vi "Set Up Dialog - Pulse.vi"() -> ()   [LabVIEW 2012]
panel:
  out "Calibration Instructions":string="1. Connect the sensor to your myDAQ as shown in the diagram above.\n\n2. Wrap the pulse sensor very snuggly around your finger with the white pad on the pad of your finger tip. You can try different fingers if the signal is not clear.\n\n3. Wait until the signal has settled then clear the chart and press \"RescaleY\" to scale the data on the chart. You should see distinct spikes with each heartbeat as pictured in Fig 1. Be patient and try to move your hand as little as possible to get a clear signal.\n\n4. Press the Calibrate button to automatically set the threshold limit to 60% of the range of the signal. You can type in your own value for the threshold if needed so that the pulse signal crosses the threshold only once per beat.\n"
  # "iWorx - Pulse - Set Up"
  # "Fig 1. Example Waveform Chart form the Pulse Data Logger VI"
  # "Pulse Sensor (PTN - 104)"
  # "iWorx"
  # "Sensor"
  # "PTN - 104"
  # "myDAQ"
  # "Computer"
  # "Adaptor"
  # "Connection Diagram"
  # "For this chart the threshold is set to 64uV, so the signal crosses the threashold once ber heartbeat."
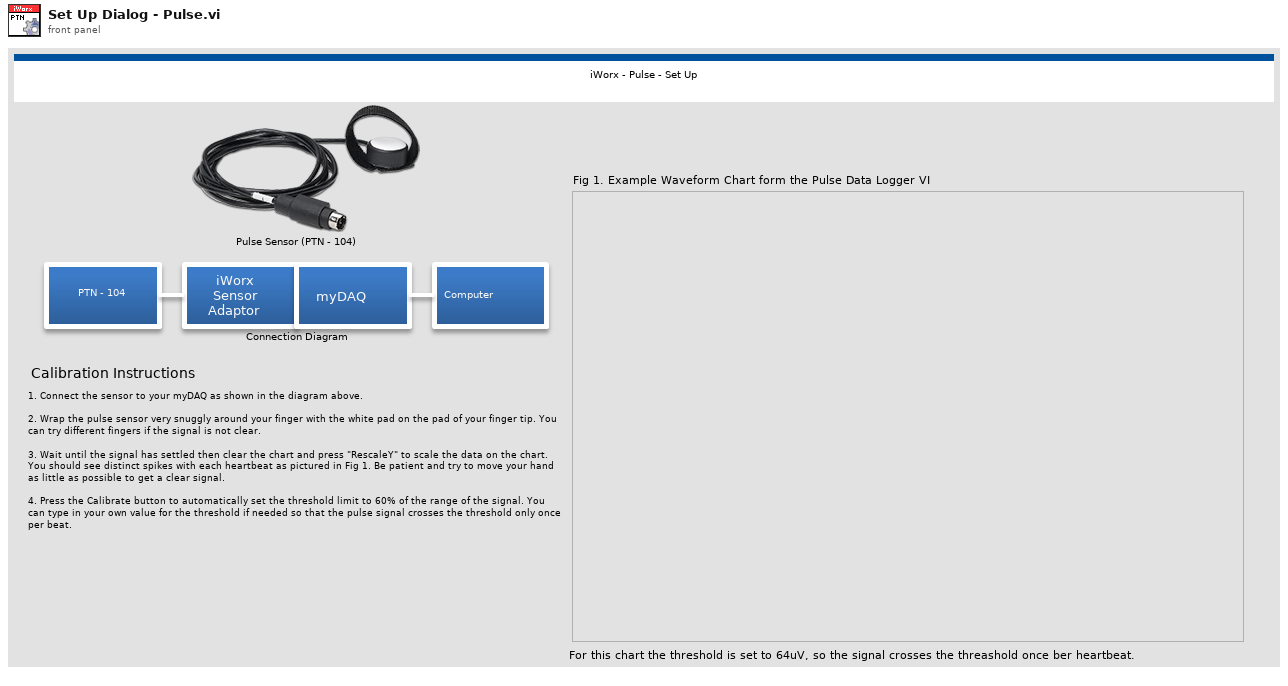
[diagram p1: front panel]
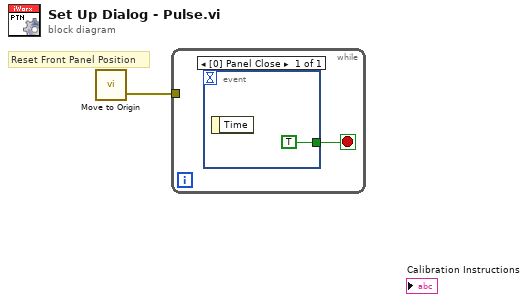
[diagram p0: block diagram]
diagram:
  # "Reset Front Panel Position"
  n1 = call "Move to Origin.vi"() -> ("Error Out"=w1:errorcluster)  [unwired: 3 in]
  n2 = while {
    tunnel: w1 -> [_]
    stop <- w2 stop-if-true
    n3 = event shown="[0] Panel Close" {
      selector: _ -> [_]
      dyn-events: _ -> [_]
      timeout: _ -> [_]
      tunnel: [TRUE] -> w2
      event Panel Close {
        n4 = event-data() -> ()  [unwired: 1 in, 1 out]
      }
    }
  }
